vi "Read Write Data.vi"(7 "Enum":T1, 8 "error in (no error)":errorcluster, 10 "Account Information":T2(array[cluster]), 11 "file path":path) -> (0 "error out":errorcluster, 2 "Array":T2(array[cluster]))   [LabVIEW 2013]
uses:
  Controls/Log Data States.ctl
  <vilib>/Utility/file.llb/Read From Spreadsheet File (string).vi
  <vilib>/Utility/file.llb/Write To Spreadsheet File (string).vi
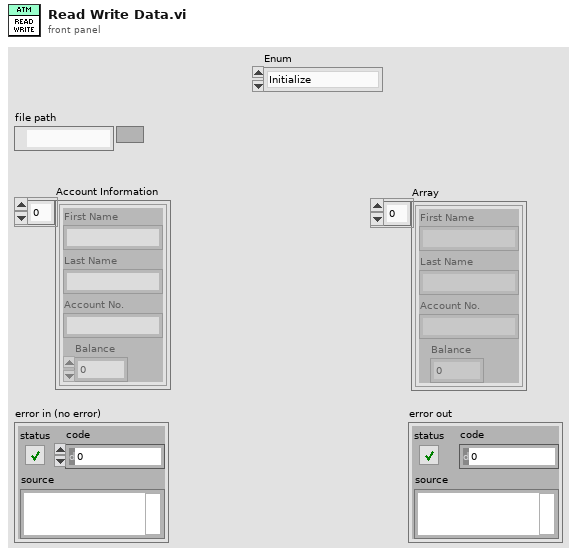
[diagram p1: front panel]
types:
  T1 = typedef "Log Data States.ctl" = enum16{"Initialize", "Read", "Write", "Stop"}
  T2 = cluster{"First Name":string, "Last Name":string, "Account No.":string, "Balance":i32}[]
  T3 = cluster{"First Name":string, "Last Name":string, "Account No.":string, "Balance":i32}
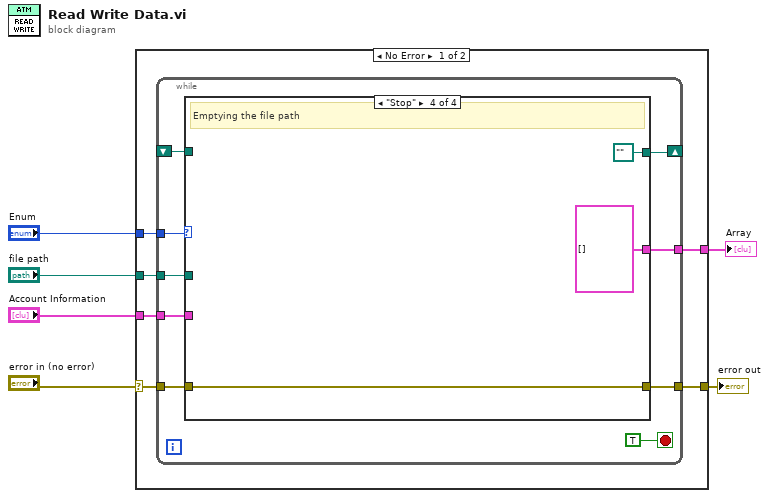
[diagram p0: block diagram]
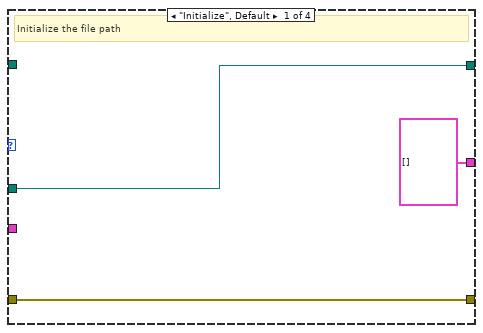
[diagram p2: hidden frame]
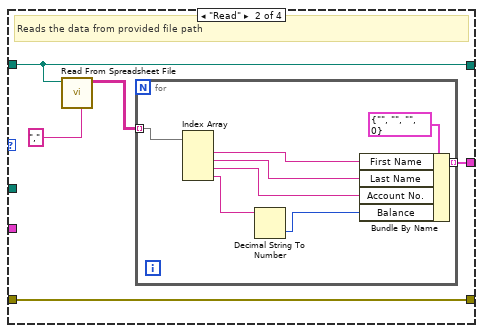
[diagram p3: hidden frame]
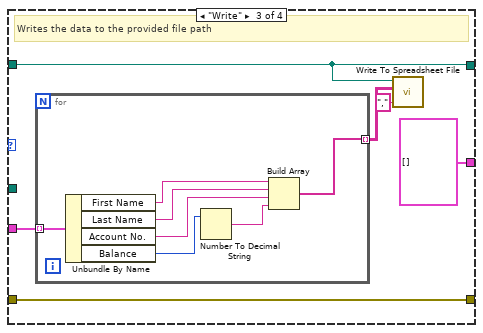
[diagram p4: hidden frame]
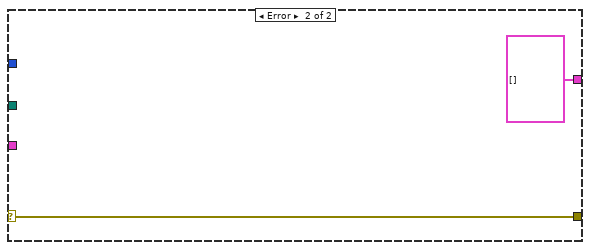
[diagram p5: hidden frame]
diagram:
  n1 = case shown="No Error" "error in (no error)" {
    selector: "error in (no error)" -> [w8 w55]
    tunnel: "Enum" -> [w12 _]
    tunnel: "file path" -> [w11 _]
    tunnel: [w10 T2 []] -> w3
    tunnel: "Account Information" -> [w9 _]
    tunnel: [w7 w55] -> w6
    frame No Error {
      n2 = while {
        tunnel: w12 -> [w20]
        tunnel: w11 -> [w19]
        shift-right: [w18] -> _
        shift-left: _ -> [w17]
        tunnel: [w16] -> w10
        tunnel: w9 -> [w15]
        tunnel: w8 -> [w14]
        tunnel: [w13] -> w7
        stop <- TRUE stop-if-true
        n3 = case shown="\"Stop\"" w20 {
          tunnel: w19 -> [w24 _ _ _]
          tunnel: [w24 w28 w43 path "" ("file path")] -> w18
          tunnel: w17 -> [_ w28 w43 _]
          tunnel: [T2 [] w26 T2 [] T2 []] -> w16
          tunnel: w15 -> [_ _ w42 _]
          tunnel: w14 -> [w22 w25 w39 w51]
          tunnel: [w22 w25 w39 w51] -> w13
          frame "Initialize", Default {
            # "Initialize the file path"
          }
          frame "Read" {
            # "Reads the data from provided file path"
            n4 = call-poly <vilib>:"Read From Spreadsheet File.vi"("delimiter (\\t)"="," ("delimiter (\\t)"), "file path (dialog if empty)"=w28) -> ("all rows"=w27:string[][])  [unwired: 5 in, 4 out]
            n5 = for {
              tunnel: w27 -> [w35] mode=indexing
              tunnel: [w37] -> w26 mode=indexing
              n6 = Index Array(array=w35) -> (element #1=w34:string, element #2=w33:string, element #3=w32:string, element #4=w31:string)  [unwired: 4 in]
              n7 = Decimal String To Number(string=w31) -> (number=w30:i32)  [unwired: 2 in, 1 out]
              n8 = Bundle By Name(cluster=T3 {"First Name"="", "Last Name"="", "Account No."="", "Balance"=0}, "First Name"=w34, "Last Name"=w33, "Account No."=w32, "Balance"=w30) -> (w37:T3)
            }
          }
          frame "Write" {
            # "Writes the data to the provided file path"
            n9 = for {
              tunnel: w42 -> [w50] mode=indexing
              tunnel: [w44] -> w41 mode=indexing
              n10 = Unbundle By Name(w50) -> ("First Name"=w49:string, "Last Name"=w48:string, "Account No."=w47:string, "Balance"=w45:i32)
              n11 = Number To Decimal String(number=w45) -> (decimal integer string=w46:string)  [unwired: 1 in]
              n12 = Build Array(w49, w48, w47, w46) -> (w44:string[])
            }
            n13 = call-poly <vilib>:"Write To Spreadsheet File.vi"("delimiter (\\t)"="," ("delimiter (\\t)"), "2D data"=w41, "file path (dialog if empty)"=w43) -> ()  [unwired: 5 in, 1 out]
          }
          frame "Stop" {
            # "Emptying the file path"
          }
        }
      }
    }
    frame Error {
    }
  }
  "error out" <- w6
  "Array" <- w3
